vi "sub-Language-get str.vi"   [LabVIEW 2011]
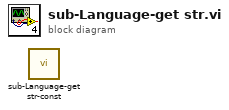
[diagram p0: block diagram]
diagram:
  n1 = call "sub-Language-get str-const.vi"() -> ()  [unwired: 1 in, 1 out]
